vi "SUB_COM9_INIT.vi"(3 "baud rate":u32=9600) -> (0 "error out":errorcluster, 1 "VISA resource name out":refnum<visa-resource-name>)   [LabVIEW 2011]
uses:
  <vilib>/Instr/_visa.llb/VISA Configure Serial Port (Instr).vi
panel:
  out "x = 0?":bool
  out "error out 3":errorcluster
  out "error out 2":errorcluster
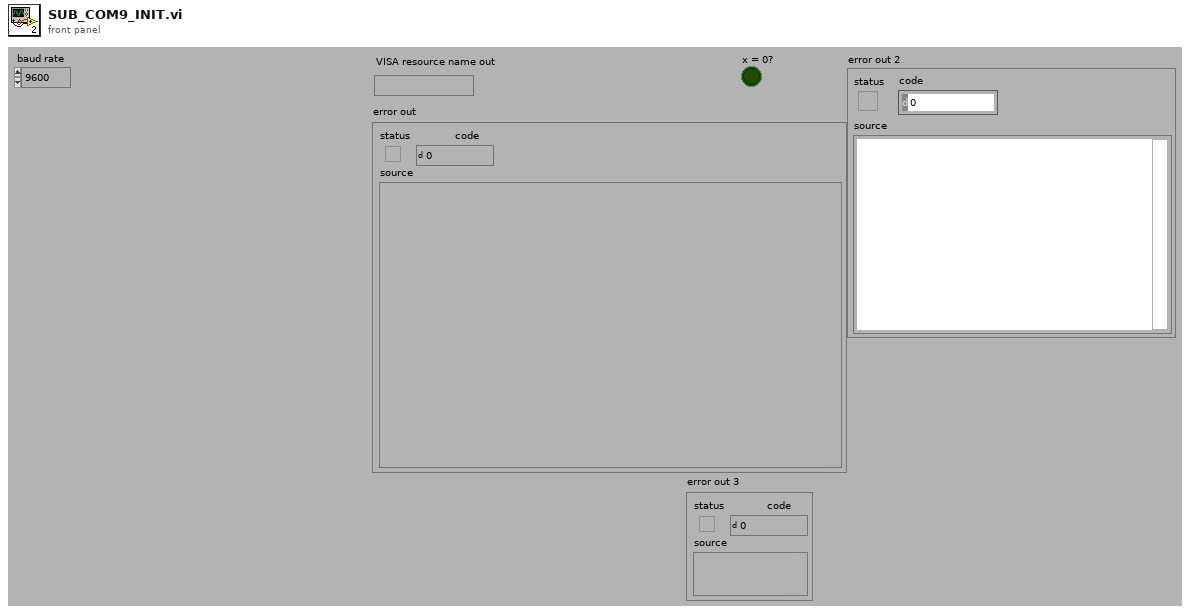
[diagram p1: front panel]
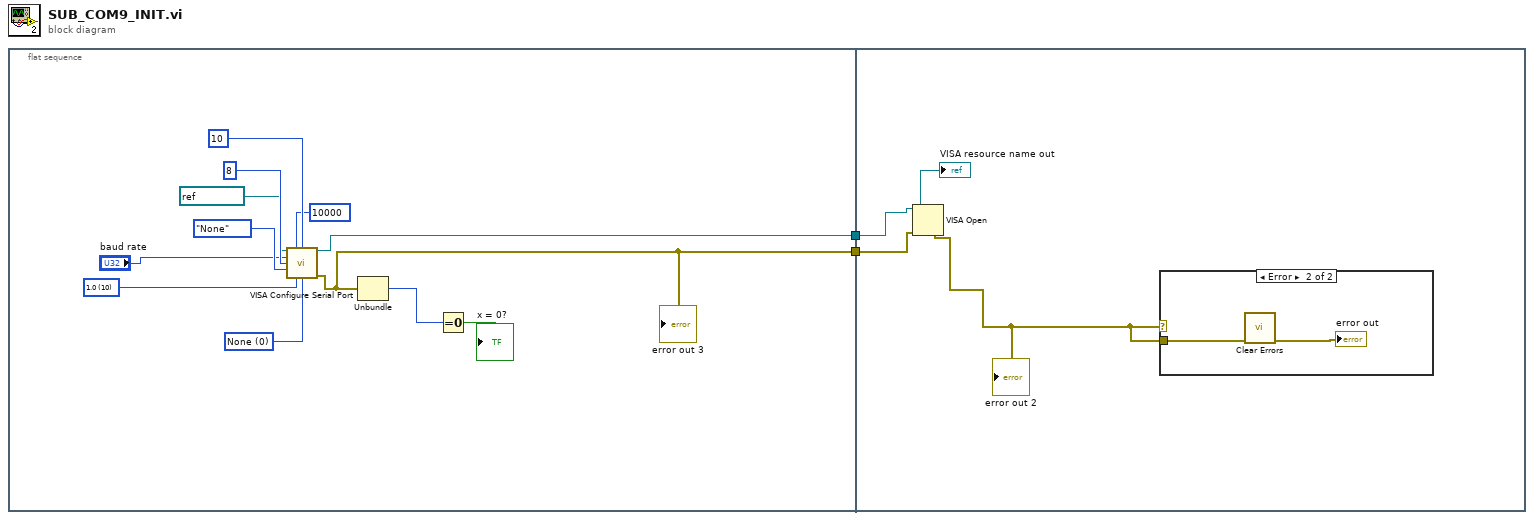
[diagram p0: block diagram]
diagram:
  n1 = flat-sequence {
    tunnel: [w14] -> w2
    tunnel: [w13] -> w1
    tunnel: w2 -> [w18]
    tunnel: w1 -> [w17]
    frame #0 {
      w5 = u16 0 items=["None", "XON/XOFF", "RTS/CTS", "XON/XOFF & RTS/CTS", "DTR/DSR", "XON/XOFF & DTR/DSR"] ("flow control (0:none)")
      w10 = u16 10 items=["1.0"=10, "1.5"=15, "2.0"=20] ("stop bits (10: 1 bit)")
      n2 = call-poly "VISA Configure Serial Port"("VISA resource name"=refnum<visa-resource-name> "COM9", "timeout (10sec)"=u32 10000, "termination char\n(0xA = '\\n' = LF)"=u8 10 ("termination char\n(0xA = '\\n' = LF)"), "baud rate (9600)"="baud rate", "data bits (8)"=u16 8, "parity (0:none)"=enum16{"None", "Odd", "Even", "Mark", "Space"}."None", "stop bits (10: 1 bit)"=w10, "flow control (0:none)"=w5) -> ("VISA resource name out"=w13:refnum<visa-resource-name>, "error out"=w14:errorcluster)  [unwired: 6 in]
      "error out 3" <- w14
      n3 = Unbundle(w14) -> ("code"=w4:i32)  [unwired: 2 out]
      n4 = Equal To 0?(x=w4) -> (x = 0?=→"x = 0?":bool)
    }
    frame #1 {
      n5 = VISA Open(error in (no error)=w18, VISA resource name=w17) -> (VISA resource name=→"VISA resource name out":refnum<visa-resource-name>, error out=w15:errorcluster)  [unwired: 3 in]
      "error out 2" <- w15
      n6 = case shown="Error" w15 {
        tunnel: w15 -> [_ w20]
        frame No Error {
        }
        frame Error {
          n7 = call <vilib>:"Clear Errors.vi"("error in (no error)"=w20) -> ("error out"=→"error out":errorcluster)  [unwired: 6 in]
        }
      }
    }
  }
